vi "Set Stage Position.vi"(3 "Position":cluster{dbl, dbl, dbl}, 4 "error in":errorcluster, 5 "VISA resource name in":refnum<visa-resource-name>) -> (1 "error out":errorcluster, 2 "VISA resource name out":refnum<visa-resource-name>)   [LabVIEW 2016]
uses:
  <vilib>/Instr/_visa.llb/VISA Configure Serial Port (Instr).vi
panel:
  out "concatenated string":string
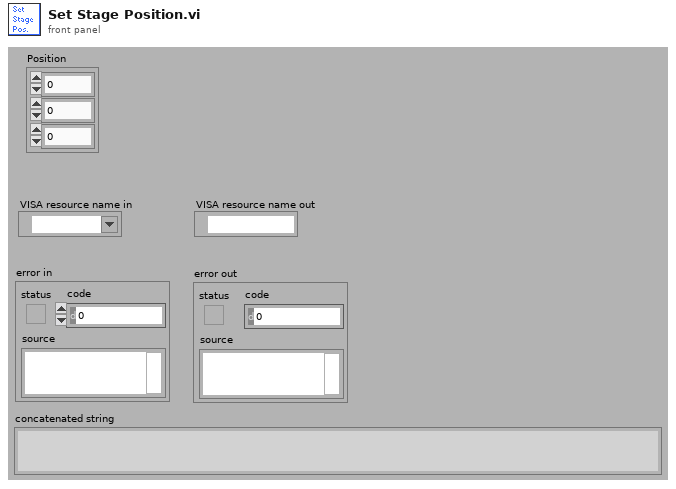
[diagram p1: front panel]
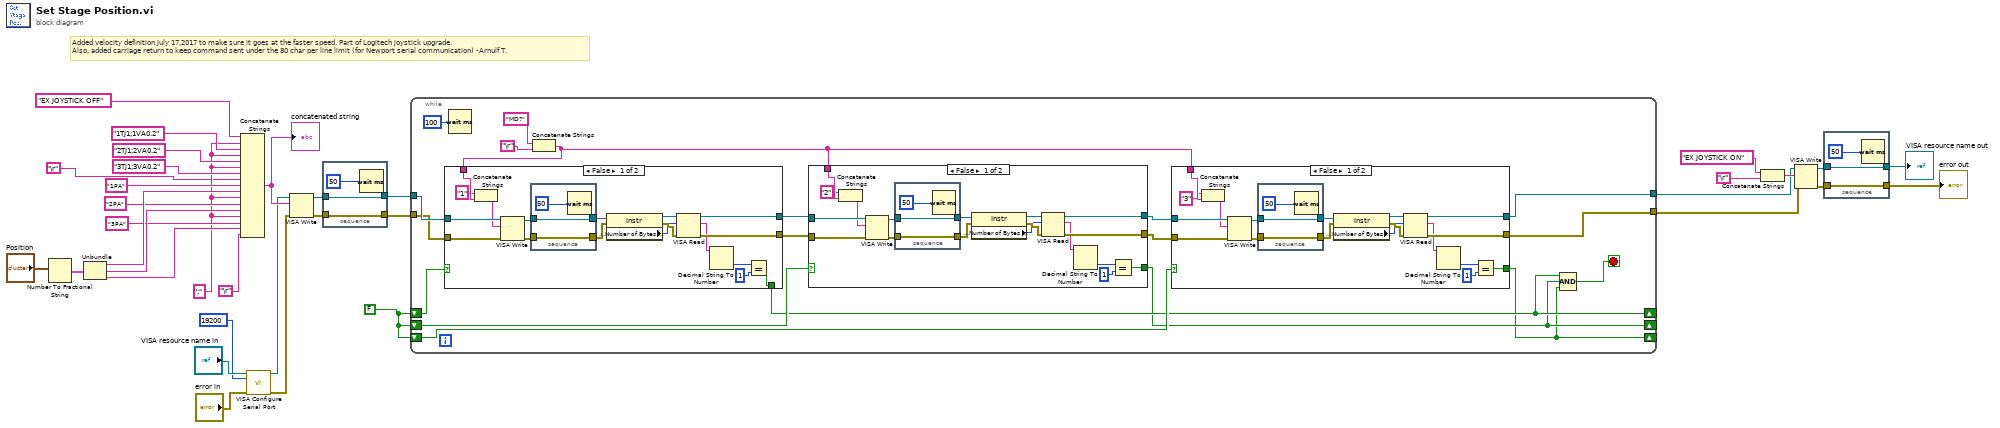
[diagram p0: block diagram]
diagram:
  w3 = FALSE
  w2 = ";"
  # "Added velocity definition July 17,2017 to make sure it goes at the faster speed. Part of Logitech joystick upgrade.\nAlso, added carriage return to keep command sent under the 80 char per line limit (for Newport serial communication) -Arnulf T."
  n1 = Number To Fractional String(number="Position") -> (F-format string=w27:cluster{string, string, string})  [unwired: 3 out]
  n2 = Unbundle(w27) -> (w26:string, w25:string, w24:string)
  n3 = Concatenate Strings("EX JOYSTICK OFF", w2, "1TJ1;1VA0.2", w2, "2TJ1;2VA0.2", w2, "3TJ1;3VA0.2", "\r", "1PA", w26, w2, "2PA", w25, w2, "3PA", w24, "\r") -> (w20:string)
  "concatenated string" <- w20
  n4 = call-poly "VISA Configure Serial Port"("VISA resource name"="VISA resource name in", "baud rate (9600)"=u32 19200, "error in (no error)"="error in") -> ("VISA resource name out"=w15:refnum<visa-resource-name>, "error out"=w14:errorcluster)  [unwired: 3 in, 8 out]
  n5 = VISA Write(VISA resource name=w15, write buffer=w20, error in (no error)=w14) -> (VISA resource name out=w19:refnum<visa-resource-name>, error out=w18:errorcluster)  [unwired: 1 out]
  n6 = stacked-sequence {
    tunnel: [w38] -> w30
    tunnel: w19 -> [w38]
    tunnel: w18 -> [w37]
    tunnel: [w37] -> w29
    frame #0 {
      n7 = Wait (ms)(milliseconds to wait=50) -> ()  [unwired: 1 out]
    }
  }
  n8 = while {
    tunnel: w30 -> [w57]
    tunnel: w29 -> [w56]
    tunnel: [w44] -> w8
    tunnel: [w43] -> w7
    shift-right: [w42] -> _
    shift-left: w3 -> [w52]
    shift-right: [w41] -> _
    shift-left: w3 -> [w46]
    shift-right: [w40] -> _
    shift-left: w3 -> [w45]
    stop <- w39 stop-if-true
    n9 = Wait (ms)(milliseconds to wait=u32 100) -> ()  [unwired: 1 out]
    n10 = Concatenate Strings("MD?" ("write buffer"), "\r") -> (w47:string)
    n11 = case shown="False" w52 {
      selector: w52 -> [_ w129]
      tunnel: w57 -> [w123 w127]
      tunnel: w56 -> [w122 w128]
      tunnel: [w121 w127] -> w51
      tunnel: [w120 w128] -> w50
      tunnel: w47 -> [w109 _]
      tunnel: [w106 w129] -> w42
      frame False {
        n12 = Concatenate Strings("1" ("string"), w109) -> (w107:string)
        n13 = VISA Write(VISA resource name=w123, write buffer=w107, error in (no error)=w122) -> (VISA resource name out=w111:refnum<visa-resource-name>, error out=w112:errorcluster)  [unwired: 1 out]
        n14 = stacked-sequence {
          tunnel: [w126] -> w113
          tunnel: w111 -> [w126]
          tunnel: w112 -> [w125]
          tunnel: [w125] -> w117
          frame #0 {
            n15 = Wait (ms)(milliseconds to wait=50) -> ()  [unwired: 1 out]
          }
        }
        n16 = property class="Instr"(reference=w113, error in=w117) -> (reference out=w114:refnum<visa-resource-name>, error out=w116:errorcluster, "Serial Settings:Number of Bytes at Serial Port"=w115:u32)
        n17 = VISA Read(VISA resource name=w114, byte count=w115, error in (no error)=w116) -> (VISA resource name out=w121:refnum<visa-resource-name>, read buffer=w110:string, error out=w120:errorcluster)  [unwired: 1 out]
        n18 = Decimal String To Number(string=w110) -> (number=w118:i32)  [unwired: 3 out]
        n19 = Equal?(x=w118, y=1) -> (x = y?=w106:bool)
      }
      frame True {
      }
    }
    n20 = case shown="False" w46 {
      selector: w46 -> [_ w105]
      tunnel: w51 -> [w99 w103]
      tunnel: w50 -> [w98 w104]
      tunnel: [w97 w103] -> w49
      tunnel: [w96 w104] -> w48
      tunnel: w47 -> [w85 _]
      tunnel: [w82 w105] -> w41
      frame False {
        n21 = Concatenate Strings("2" ("string"), w85) -> (w83:string)
        n22 = VISA Write(VISA resource name=w99, write buffer=w83, error in (no error)=w98) -> (VISA resource name out=w87:refnum<visa-resource-name>, error out=w88:errorcluster)  [unwired: 1 out]
        n23 = stacked-sequence {
          tunnel: [w102] -> w89
          tunnel: w87 -> [w102]
          tunnel: w88 -> [w101]
          tunnel: [w101] -> w93
          frame #0 {
            n24 = Wait (ms)(milliseconds to wait=50) -> ()  [unwired: 1 out]
          }
        }
        n25 = property class="Instr"(reference=w89, error in=w93) -> (reference out=w90:refnum<visa-resource-name>, error out=w92:errorcluster, "Serial Settings:Number of Bytes at Serial Port"=w91:u32)
        n26 = VISA Read(VISA resource name=w90, byte count=w91, error in (no error)=w92) -> (VISA resource name out=w97:refnum<visa-resource-name>, read buffer=w86:string, error out=w96:errorcluster)  [unwired: 1 out]
        n27 = Decimal String To Number(string=w86) -> (number=w94:i32)  [unwired: 3 out]
        n28 = Equal?(x=w94, y=1) -> (x = y?=w82:bool)
      }
      frame True {
      }
    }
    n29 = case shown="False" w45 {
      selector: w45 -> [_ w81]
      tunnel: w49 -> [w75 w79]
      tunnel: w48 -> [w74 w80]
      tunnel: [w73 w79] -> w44
      tunnel: [w72 w80] -> w43
      tunnel: w47 -> [w61 _]
      tunnel: [w58 w81] -> w40
      frame False {
        n30 = Concatenate Strings("3" ("string"), w61) -> (w59:string)
        n31 = VISA Write(VISA resource name=w75, write buffer=w59, error in (no error)=w74) -> (VISA resource name out=w63:refnum<visa-resource-name>, error out=w64:errorcluster)  [unwired: 1 out]
        n32 = stacked-sequence {
          tunnel: [w78] -> w65
          tunnel: w63 -> [w78]
          tunnel: w64 -> [w77]
          tunnel: [w77] -> w69
          frame #0 {
            n33 = Wait (ms)(milliseconds to wait=50) -> ()  [unwired: 1 out]
          }
        }
        n34 = property class="Instr"(reference=w65, error in=w69) -> (reference out=w66:refnum<visa-resource-name>, error out=w68:errorcluster, "Serial Settings:Number of Bytes at Serial Port"=w67:u32)
        n35 = VISA Read(VISA resource name=w66, byte count=w67, error in (no error)=w68) -> (VISA resource name out=w73:refnum<visa-resource-name>, read buffer=w62:string, error out=w72:errorcluster)  [unwired: 1 out]
        n36 = Decimal String To Number(string=w62) -> (number=w70:i32)  [unwired: 3 out]
        n37 = Equal?(x=w70, y=1) -> (x = y?=w58:bool)
      }
      frame True {
      }
    }
    n38 = Compound Arithmetic op=AND(w42, w41, w40) -> (w39:bool)
  }
  n39 = Concatenate Strings("EX JOYSTICK ON" ("write buffer"), "\r") -> (w13:string)
  n40 = VISA Write(VISA resource name=w8, write buffer=w13, error in (no error)=w7) -> (VISA resource name out=w10:refnum<visa-resource-name>, error out=w11:errorcluster)  [unwired: 1 out]
  n41 = stacked-sequence {
    tunnel: [w132] -> w32
    tunnel: w10 -> [w132]
    tunnel: w11 -> [w131]
    tunnel: [w131] -> w31
    frame #0 {
      n42 = Wait (ms)(milliseconds to wait=50) -> ()  [unwired: 1 out]
    }
  }
  "VISA resource name out" <- w32
  "error out" <- w31
